vi "Main Graphics Loop.vi"(8 "error in (no error)":errorcluster, 11 "Application in":refnum<class "Application.lvclass">) -> (0 "error out":errorcluster)   [LabVIEW 2021, in "Application.lvclass"]
uses:
  Application.lvclass
  Application.lvclass/Application.ctl
  GameEl_class/GameEl.lvclass
  Board Game_class/Board Game.lvclass
  Board Game_class/Board Game.lvclass/Board Game.ctl
  Board Game_class/Read Board Game Ref.vi
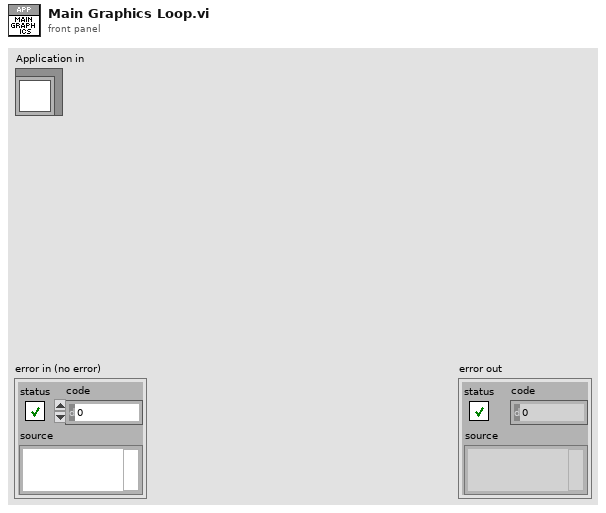
[diagram p1: front panel]
types:
  T1 = cluster{"GameEl":refnum<class "GameEl.lvclass">, "Board Game in":refnum<class "Board Game.lvclass">}
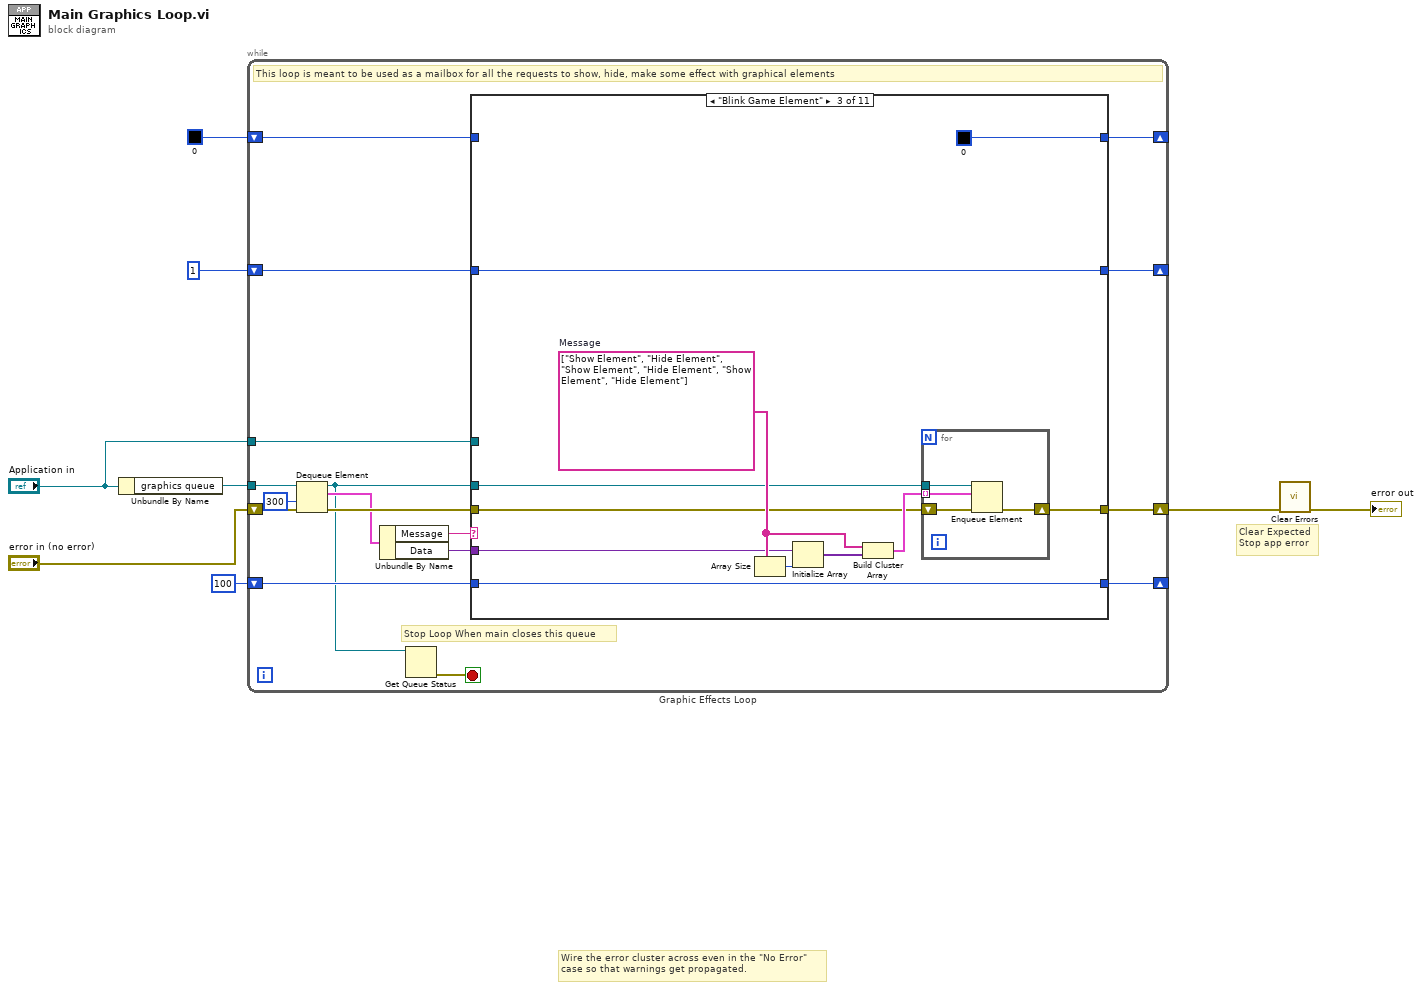
[diagram p0: block diagram]
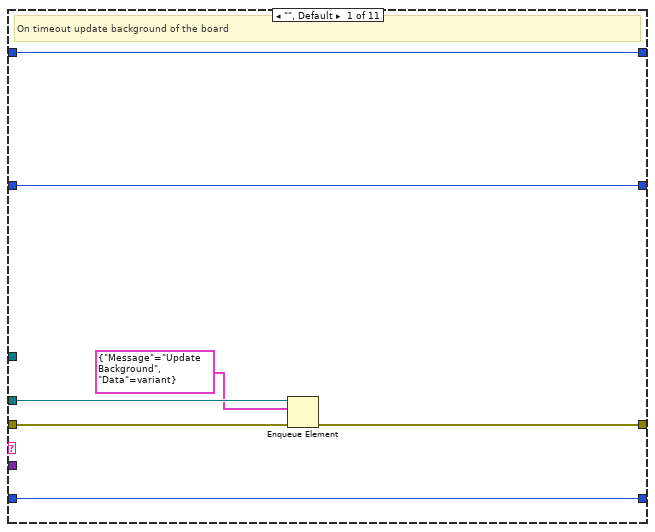
[diagram p2: hidden frame]
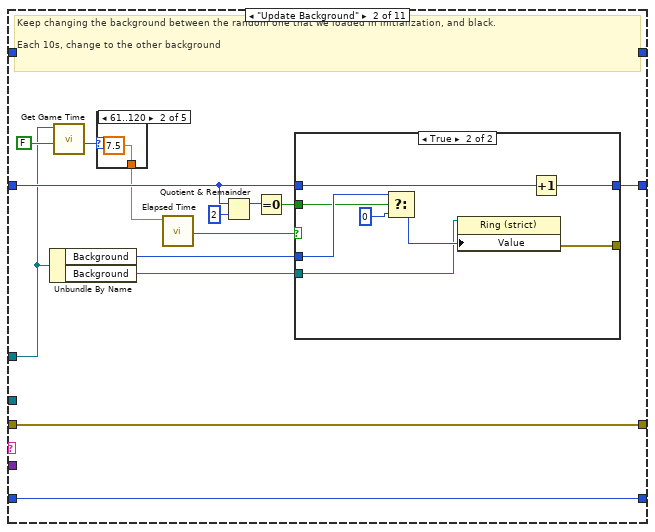
[diagram p3: hidden frame]
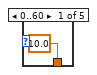
[diagram p4: hidden frame]
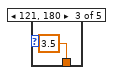
[diagram p5: hidden frame]
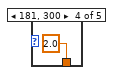
[diagram p6: hidden frame]
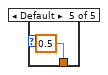
[diagram p7: hidden frame]
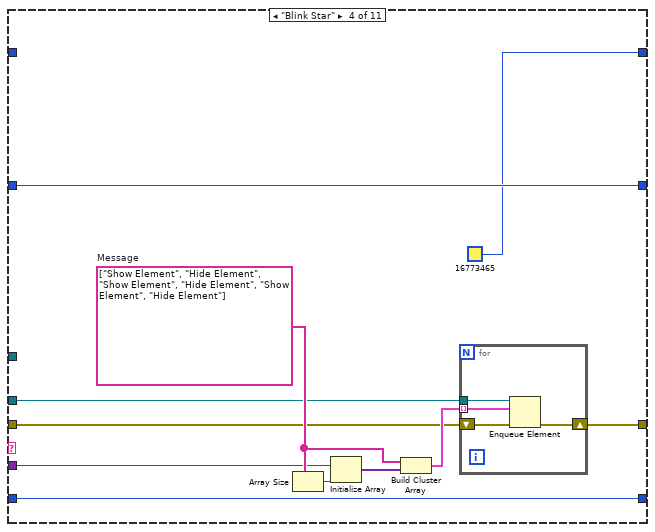
[diagram p9: hidden frame]
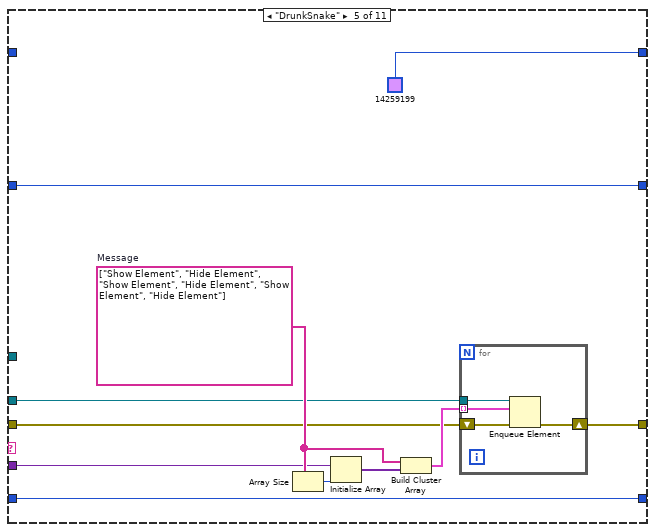
[diagram p10: hidden frame]
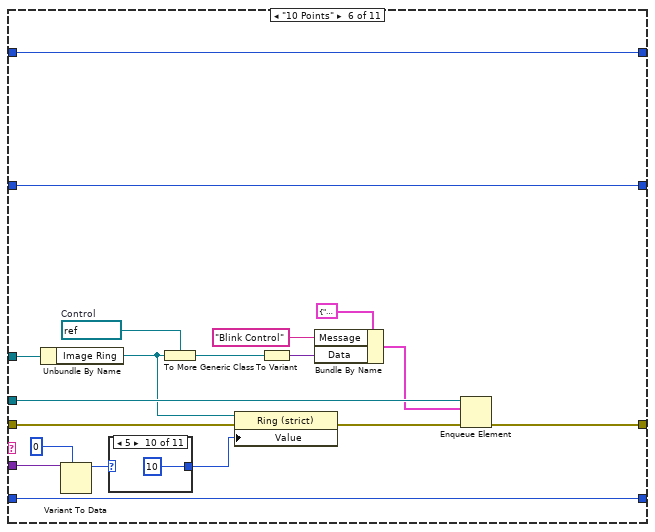
[diagram p11: hidden frame]
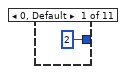
[diagram p12: hidden frame]
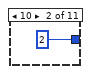
[diagram p13: hidden frame]
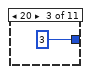
[diagram p14: hidden frame]
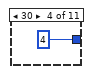
[diagram p15: hidden frame]
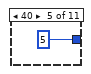
[diagram p16: hidden frame]
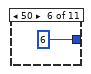
[diagram p17: hidden frame]
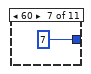
[diagram p18: hidden frame]
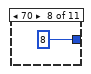
[diagram p19: hidden frame]
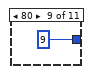
[diagram p20: hidden frame]
diagram:
  # "Clear Expected\nStop app error"
  # "Wire the error cluster across even in the \"No Error\"\ncase so that warnings get propagated."
  n1 = Unbundle By Name("Application in") -> ("graphics queue"=w8:refnum<queue>)
  n2 = while "Graphic Effects Loop" {
    tunnel: w8 -> [w24]
    shift-right: [w21] -> w4
    shift-left: "error in (no error)" -> [w23]
    tunnel: "Application in" -> [w17]
    shift-right: [w15] -> _
    shift-left: 100 ("timeout in ms (-1)") -> [w16]
    shift-right: [w13] -> _
    shift-left: u32 0 ("Colour") -> [w14]
    shift-right: [w9] -> _
    shift-left: 1 ("Numeric") -> [w10]
    stop <- w25 stop-if-true
    # "Stop Loop When main closes this queue"
    # "This loop is meant to be used as a mailbox for all the requests to show, hide, make some effect with graphical elements"
    n3 = Dequeue Element(queue=w24, timeout in ms (-1)=300, error in (no error)=w23) -> (queue out=w11:refnum<queue>, element=w20:cluster{"Message":string, "Data":variant}, error out=w22:errorcluster)  [unwired: 1 out]
    n4 = Unbundle By Name(w20) -> ("Message"=w19:string, "Data"=w18:variant)
    n5 = Get Queue Status(queue=w11) -> (error out=w25:errorcluster)  [unwired: 2 in, 7 out]
    n6 = case shown="\"Blink Game Element\"" w19 {
      tunnel: w22 -> [w32 w37 w65 w79 w93 w122 w144 w158 w171 w186 w199]
      tunnel: [w29 w37 w65 w79 w93 w121 w143 w153 w165 w180 w194] -> w21
      tunnel: w18 -> [_ _ w64 w78 w92 w110 w140 w157 w172 w187 w198]
      tunnel: w17 -> [_ w35 _ _ _ w119 _ _ _ _ _]
      tunnel: w16 -> [w31 w47 w71 w85 w99 w115 w142 w159 w174 w189 w200]
      tunnel: [w31 w47 w71 w85 w99 w115 w142 w159 w174 w189 w200] -> w15
      tunnel: w14 -> [w30 w46 _ _ _ w105 w135 w150 w161 w176 w191]
      tunnel: [w30 w46 u32 0 ("Colour") u32 16773465 ("Colour") u32 14259199 ("Colour") w105 w135 w150 w161 w176 w191] -> w13
      tunnel: w11 -> [w28 _ w66 w80 w94 w120 w141 _ _ _ _]
      tunnel: w10 -> [w26 w39 w62 w77 w90 w104 w134 w149 w160 w175 w190]
      tunnel: [w26 w41 w62 w77 w90 w104 w134 w149 w160 w175 w190] -> w9
      frame "", Default {
        # "On timeout update background of the board"
        n7 = Enqueue Element(queue=w28, element=cluster{"Message":string, "Data":variant} {"Message"="Update Background", "Data"=variant}, error in (no error)=w32) -> (error out=w29:errorcluster)  [unwired: 1 in, 2 out]
      }
      frame "Update Background" {
        # "Keep changing the background between the random one that we loaded in initialization, and black. \n\nEach 10s, change to the other background"
        n8 = Unbundle By Name(w35) -> ("Background"=w38:u16, "Background"=w40:refnum<vi>)
        n9 = call "Get Game Time.vi"("Pause/Resume"=FALSE, "Application in"=w35) -> ("Elapsed"=w34:u32)  [unwired: 7 in, 2 out]
        n10 = case shown="61..120" w34 {
          tunnel: [10.0 ("Time Target (s)") 7.5 ("Time Target (s)") 3.5 ("Time Target (s)") 2.0 ("Time Target (s)") 0.5 ("Time Target (s)")] -> w33
          frame 0..60 {
          }
          frame 61..120 {
          }
          frame 121, 180 {
          }
          frame 181, 300 {
          }
          frame Default {
          }
        }
        n11 = call "Elapsed Time"("Time Target (s)"=w33) -> ("Time has Elapsed"=w45:bool)  [unwired: 11 in, 7 out]
        n12 = Quotient & Remainder(x=w39, y=2) -> (x-y*floor(x/y)=w44:i32)  [unwired: 1 out]
        n13 = Equal To 0?(x=w44) -> (x = 0?=w43:bool)
        n14 = case shown="True" w45 {
          tunnel: [_ w61] -> _
          tunnel: w43 -> [_ w54]
          tunnel: w39 -> [w53 w58]
          tunnel: [w53 w57] -> w41
          tunnel: w40 -> [_ w56]
          tunnel: w38 -> [_ w55]
          frame False {
          }
          frame True {
            n15 = Select(t=w55, s=w54, f=u16 0) -> (s? t:f=w60:u16)
            n16 = property class="Ring (strict)"(reference=w56, "Value"=w60) -> (error out=w61:errorcluster)  [unwired: 1 in, 1 out]
            n17 = Increment(x=w58) -> (x+1=w57:i32)
          }
        }
      }
      frame "Blink Game Element" {
        w69 = string[] ["Show Element", "Hide Element", "Show Element", "Hide Element", "Show Element", "Hide Element"]  # Message
        n18 = Array Size(array=w69) -> (size(s)=w70:i32)
        n19 = Initialize Array(w64, w70) -> (w68:variant[])
        n20 = Build Cluster Array(w69, w68) -> (w67:cluster{"String":string, "Data":variant}[])
        n21 = for {
          tunnel: w66 -> [w73]
          shift-right: [w74] -> _
          shift-left: _ -> [w75]
          tunnel: w67 -> [w72] mode=indexing
          n22 = Enqueue Element(queue=w73, element=w72, error in (no error)=w75) -> (error out=w74:errorcluster)  [unwired: 1 in, 2 out]
        }
      }
      frame "Blink Star" {
        w83 = string[] ["Show Element", "Hide Element", "Show Element", "Hide Element", "Show Element", "Hide Element"]  # Message
        n23 = Array Size(array=w83) -> (size(s)=w84:i32)
        n24 = Initialize Array(w78, w84) -> (w82:variant[])
        n25 = Build Cluster Array(w83, w82) -> (w81:cluster{"String":string, "Data":variant}[])
        n26 = for {
          tunnel: w80 -> [w87]
          shift-right: [w88] -> _
          shift-left: _ -> [w89]
          tunnel: w81 -> [w86] mode=indexing
          n27 = Enqueue Element(queue=w87, element=w86, error in (no error)=w89) -> (error out=w88:errorcluster)  [unwired: 1 in, 2 out]
        }
      }
      frame "DrunkSnake" {
        w97 = string[] ["Show Element", "Hide Element", "Show Element", "Hide Element", "Show Element", "Hide Element"]  # Message
        n28 = Array Size(array=w97) -> (size(s)=w98:i32)
        n29 = Initialize Array(w92, w98) -> (w96:variant[])
        n30 = Build Cluster Array(w97, w96) -> (w95:cluster{"String":string, "Data":variant}[])
        n31 = for {
          tunnel: w94 -> [w101]
          shift-right: [w102] -> _
          shift-left: _ -> [w103]
          tunnel: w95 -> [w100] mode=indexing
          n32 = Enqueue Element(queue=w101, element=w100, error in (no error)=w103) -> (error out=w102:errorcluster)  [unwired: 1 in, 2 out]
        }
      }
      frame "10 Points" {
        w113 = refnum<vi> refnum  # Control
        n33 = Unbundle By Name(w119) -> ("Image Ring"=w108:refnum<vi>)
        n34 = Variant To Data(type=u16 0, Variant=w110) -> (data=w107:u16)  [unwired: 1 in, 1 out]
        n35 = case shown="5" w107 {
          tunnel: [u16 2 ("Value") u16 2 ("Value") u16 3 ("Value") u16 4 ("Value") u16 5 ("Value") u16 6 ("Value") u16 7 ("Value") u16 8 ("Value") u16 9 ("Value") u16 10 ("Value") u16 11 ("Value")] -> w106
          frame 0, Default {
          }
          frame 10 {
          }
          frame 20 {
          }
          frame 30 {
          }
          frame 40 {
          }
          frame 50 {
          }
          frame 60 {
          }
          frame 70 {
          }
          frame 80 {
          }
          frame 5 {
          }
          frame 6 {
          }
        }
        n36 = To More Generic Class(target class=w113, reference=w108) -> (generic class reference=w114:refnum<vi>)
        n37 = property class="Ring (strict)"(reference=w108, error in=w122, "Value"=w106) -> (error out=w111:errorcluster)  [unwired: 1 out]
        n38 = To Variant(anything=w114) -> (Variant=w117:variant)
        n39 = Bundle By Name(cluster=cluster{"Message":string, "Data":variant} {"Message"="", "Data"=variant} ("element"), "Message"="Blink Control", "Data"=w117) -> (w112:cluster{"Message":string, "Data":variant})
        n40 = Enqueue Element(queue=w120, element=w112, error in (no error)=w111) -> (error out=w121:errorcluster)  [unwired: 1 in, 2 out]
      }
      frame "Blink Control" {
        w138 = string[] ["Show Control", "Hide Control", "Show Control", "Hide Control", "Show Control", "Hide Control"]  # Message
        n41 = Array Size(array=w138) -> (size(s)=w139:i32)
        n42 = Initialize Array(w140, w139) -> (w137:variant[])
        n43 = Build Cluster Array(w138, w137) -> (w136:cluster{"String":string, "Data":variant}[])
        n44 = for {
          tunnel: w141 -> [w146]
          shift-right: [w147] -> w143
          shift-left: w144 -> [w148]
          tunnel: w136 -> [w145] mode=indexing
          n45 = Enqueue Element(queue=w146, element=w145, error in (no error)=w148) -> (error out=w147:errorcluster)  [unwired: 1 in, 2 out]
        }
      }
      frame "Show Control" {
        w156 = refnum<vi> refnum  # Control
        n46 = Variant To Data(error in=w158, type=w156, Variant=w157) -> (data=w152:refnum<vi>, error out=w154:errorcluster)
        n47 = property class="Ctl"(reference=w152, error in=w154, "Visible"=TRUE) -> (error out=w153:errorcluster)  [unwired: 1 out]
        n48 = Wait (ms)(milliseconds to wait=u32 125) -> ()  [unwired: 1 out]
      }
      frame "Show Element" {
        n49 = Variant To Data(error in=w171, type=T1 {"GameEl"=refnum, "Board Game in"=refnum}, Variant=w172) -> (data=w169:T1, error out=w168:errorcluster)
        n50 = Unbundle By Name(w169) -> ("GameEl"=w164:refnum<class "GameEl.lvclass">, "Board Game in"=w163:refnum<class "Board Game.lvclass">)
        n51 = property class="Board Game"(reference=w163, error in=w168) -> (error out=w166:errorcluster, "dataAccess:Board Game Ref"=w167:refnum<vi>)  [unwired: 1 out]
        n52 = call "Make Element Blink.vi"("Colour"=w161, "Board Game in"=w163, "GameEl in"=w164) -> ("Current Values"=w162:u32[][])  [unwired: 5 in, 3 out]
        n53 = property class="Arr (strict)"(reference=w167, error in=w166, "Value"=w162) -> (error out=w165:errorcluster)  [unwired: 1 out]
        n54 = Wait (ms)(milliseconds to wait=u32 200) -> ()  [unwired: 1 out]
      }
      frame "Hide Element" {
        n55 = Variant To Data(error in=w186, type=T1 {"GameEl"=refnum, "Board Game in"=refnum}, Variant=w187) -> (data=w184:T1, error out=w183:errorcluster)
        n56 = Unbundle By Name(w184) -> ("GameEl"=w179:refnum<class "GameEl.lvclass">, "Board Game in"=w178:refnum<class "Board Game.lvclass">)
        n57 = property class="Board Game"(reference=w178, error in=w183) -> (error out=w181:errorcluster, "dataAccess:Board Game Ref"=w182:refnum<vi>)  [unwired: 1 out]
        n58 = call "Make Element Blink.vi"("Colour"=w176, "Board Game in"=w178, "GameEl in"=w179) -> ("Blink Values"=w177:u32[][])  [unwired: 5 in, 3 out]
        n59 = property class="Arr (strict)"(reference=w182, error in=w181, "Value"=w177) -> (error out=w180:errorcluster)  [unwired: 1 out]
        n60 = Wait (ms)(milliseconds to wait=u32 200) -> ()  [unwired: 1 out]
      }
      frame "Hide Control" {
        w197 = refnum<vi> refnum  # Control
        n61 = Variant To Data(error in=w199, type=w197, Variant=w198) -> (data=w193:refnum<vi>, error out=w195:errorcluster)
        n62 = property class="Ctl"(reference=w193, error in=w195, "Visible"=FALSE) -> (error out=w194:errorcluster)  [unwired: 1 out]
        n63 = Wait (ms)(milliseconds to wait=u32 125) -> ()  [unwired: 1 out]
      }
    }
  }
  n64 = call <vilib>:"Clear Errors.vi"("error in (no error)"=w4) -> ("error out"=→"error out":errorcluster)  [unwired: 5 in, 1 out]
